vi "Pass Allowed Message.vi"   [LabVIEW 2017, in "_csmlite.lvlib"]
uses:
  _csmlite.lvlib
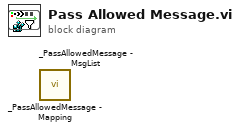
[diagram p0: block diagram]
diagram:
  n1 = call "_PassAllowedMessage - Mapping.vi"() -> ()  [unwired: 9 in, 1 out]
  n2 = call "_PassAllowedMessage - MsgList.vi"() -> ()  [unwired: 9 in, 1 out]
